vi "WK6440B_CommandsGlobal.vi"() -> ()   [LabVIEW 2019, in "WK6440B.lvclass"]
uses:
  WK6440B.lvclass
panel:
  in  "WayneKerr 6440B GPIB Setup":T1={"Instrument name"="WayneKerr 6440B", "Instrument type"=1, "Command \"Initialise LCR\""=":MEAS:EQU-CCT %s; :MEAS:FREQ %d; :MEAS:LEV %1.2fV; :MEAS; :MEAS:RANGE 5; :MEAS:SPEED MED; :MEAS:FUNC:C; :TRIG;", "Command \"OC Trim\""=":CAL; :CAL:OC-TRIM 1;", "Command \"LCR Readout\""="TRIG;"} {"Instrument type" items=["Supply", "LCR"]}
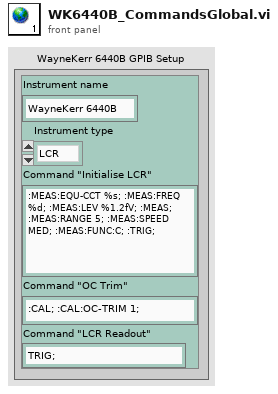
[diagram p1: front panel]
types:
  T1 = cluster{"Instrument name":string, "Instrument type":u16, "Command \"Initialise LCR\"":string, "Command \"OC Trim\"":string, "Command \"LCR Readout\"":string}
diagram:
